vi "TDC_DAQV27_Paralled_muon.vi"(7 "address":string="192.168.10.20", 8 "error in (no error)":errorcluster, 9 "stop":bool, 10 "save data":bool=TRUE, 11 "SMA mode":bool=TRUE) -> (0 "error out 3":errorcluster, 2 "appended path":path=path "G:/tdc/2017/test_20250117_110508.dat", 3 "rate":dbl=15.409526451492772)   [LabVIEW 2017]
uses:
  <vilib>/Utility/file.llb/Write Delimited Spreadsheet (DBL).vi
  <vilib>/Utility/file.llb/Write Delimited Spreadsheet (I64).vi
panel:
  in  "timeot":dbl
  out "nearest integer value":dbl
  out "Out":u8=1 format="%.0x"
  out "fine 4":u64=243508331 format="%x"
  out "fine 3":u64=243508331 format="%x"
  out "channel number 2":u64 format="%x"
  out "substring 3":string
  out "fine 2":u64=243508331 format="%x"
  out "substring 2":string
  out "substring":string
  in  "gps":bool
  out "Year":string="2025"
  in  "factor":i32=128
  in  "displayCR":bool=TRUE
  in  "Counter Setting":dbl=100000.0 format="%#_13g"
  in  "replace dat":bool
  in  "append csv":bool=TRUE
  out "element":string
  out "fine":u64=416 format="%x"
  in  "UDP Config":bool=TRUE
  in  "data  path":path=path "G:/tdc/2017/data"
  out "cal 2":u64[](graph)
  in  "Thresholds (mV)":dbl[](array[numeric])=[580.0, 580.0, 580.0, 580.0, 600.0, 600.0, 600.0, 600.0, 580.0, 580.0, 600.0, 600.0, 600.0, 600.0, 600.0, 600.0, 580.0, 580.0, 600.0, 600.0, 600.0, 600.0, 600.0, 600.0, 580.0, 580.0, 600.0, 600.0, 600.0, 600.0, 600.0, 600.0, 600.0, 600.0, 600.0, 600.0, 600.0, 600.0, 600.0, 600.0, 600.0, 600.0, 600.0, 600.0, 600.0, 600.0, 600.0, 600.0, 600.0, 600.0, 600.0, 600.0, 600.0, 600.0, 600.0, 600.0, 600.0, 600.0, 600.0, 600.0, 600.0, 600.0, 600.0, 600.0]
  out "error out 2":errorcluster={"status"=TRUE, "code"=1, "source"="Dequeue Element in TDC_DAQV27_Paralled_muon.vi"}
  in  "display":bool=TRUE
  in  "Thresholds":dbl=8191.0
  in  "one key for threshold":bool=TRUE
  in  "RST":bool
  in  "通道数量":i32=128
  out "Cal Table":u32[](array[numeric])=[5700, 5700, 0, 0, 0, 0, 0, 0, 0, 0, 0, 0, 0, 0, 0, 0, 0, 0, 0, 0, 0, 0, 0, 0, 0, 0, 0, 0, 0, 0, 0, 0, 0, 0, 0, 0, 0, 0, 0, 0, 0, 0, 0, 0, 0, 0, 0, 0, 0, 0, 0, 0, 0, 0, 0, 0, 0, 0, 0, 0, 0, 0, 0, 0, 0, 0, 0, 0, 0, 0, 0, 0, 0, 0, 0, 0, 0, 0, 0, 0, 0, 0, 0, 0, 0, 0, 0, 0, 0, 0, 0, 0, 0, 0, 0, 0, 0, 0, 0, 0, 0, 0, 0, 0, 0, 0, 0, 0, 0, 0, 0, 0, 0, 0, 0, 0, 0, 0, 0, 0, 0, 0, 0, 0, 0, 0, 0, 0]
  in  "channel for cal":i32=1
  out "channel number":u64
  in  "bytes to read":i32=320
  out "Calibration Counter":i32=5699
  out "Event index":i32=97959
  out "cal":u32[](graph)=[0, 0, 0, 0, 0, 0, 0, 0, 0, 0, 0, 0, 0, 0, 0, 0, 0, 0, 0, 0, 0, 0, 0, 0, 0, 0, 0, 0, 0, 0, 0, 0, 0, 0, 0, 0, 0, 0, 0, 0, 0, 0, 0, 0, 0, 0, 0, 0, 0, 0, 0, 0, 0, 0, 0, 0, 0, 0, 0, 0, 0, 0, 0, 0, 0, 0, 0, 0, 0, 0, 0, 0, 0, 0, 0, 0, 0, 0, 0, 0, 0, 0, 0, 0, 0, 0, 0, 0, 0, 0, 0, 0, 0, 0, 0, 0, 0, 0, 0, 0, 0, 0, 0, 0, 0, 0, 0, 0, 0, 0, 0, 0, 0, 0, 0, 0, 0, 0, 0, 0, 0, 0, 0, 0, 0, 0, 0, 0, 0, 0, 0, 0, 0, 0, 0, 0, 0, 0, 0, 0, 0, 0, 0, 0, 0, 0, 0, 0, 0, 0, 0, 0, 0, 0, 0, 0, 0, 0, 0, 0, 0, 0, 0, 0, 0, 0, 0, 0, 0, 0, 0, 0, 0, 0, 0, 0, 0, 0, 0, 0, 0, 0, 0, 0, 0, 0, 0, 0, 0, 0, 0, 0, 0, 0, 0, 0, 0, 0, 0, 0, 0, 0, 0, 0, 0, 0, 0, 0, 0, 0, 0, 0, 0, 0, 0, 0, 0, 0, 0, 0, 0, 0, 0, 0, 0, 0, 0, 0, 15, 4, 8, 11, 19, 27, 12, 4, 29, 16, 7, 12, 3, 18, 8, 6, 6, 7, 3, 6, 4, 22, 0, 10, 13, 5, 6, 5, 8, 11, 3, 15, 13, 3, 10, 19, 16, 9, 12, 2, 11, 3, 19, 2, 4, 11, 12, 2, 0, 0, 0, 0, 0, 0, 0, 0, 0, 0, 0, 0, 0, 0, 0, 0, 0, 0, 0, 0, 0, 0, 0, 0, 17, 11, 8, 5, 6, 2, 5, 3, 1, 0, 0, 0, 0, 0, 1, 5, 3, 3, 2, 0, 0, 0, 0, 0, 0, 0, 1, 0, 2, 6, 6, 10, 9, 10, 15, 8, 9, 12, 7, 6, 9, 16, 13, 16, 23, 9, 3, 5, 21, 9, 15, 40, 30, 8, 12, 2, 10, 5, 7, 12, 16, 10, 5, 11, 11, 18, 7, 12, 15, 10, 9, 13, 17, 14, 4, 6, 15, 5, 7, 2, 9, 4, 9, 6, 26, 8, 5, 14, 10, 6, 6, 10, 16, 7, 12, 10, 20, 14, 25, 8, 1, 4, 2, 14, 3, 8, 6, 5, 10, 12, 3, 6, 5, 11, 8, 17, 3, 9, 5, 0, 0, 0, 0, 0, 0, 0, 0, 0, 0, 0, 0, 0, 0, 0, 0, 0, 0, 0, 0, 0, 0, 0, 0, 5, 6, 15, 12, 7, 9, 5, 10, 4, 1, 1, 0, 0, 0, 0, 0, 0, 0, 0, 0, 0, 0, 0, 0, 0, 0, 0, 0, 0, 0, 0, 0, 3, 3, 8, 10, 10, 4, 17, 8, 4, 3, 12, 10, 26, 10, 14, 9, 31, 11, 54, 7, 12, 8, 6, 14, 7, 7, 17, 29, 8, 22, 3, 11, 12, 7, 13, 7, 5, 8, 1, 10, 10, 14, 15, 11, 8, 13, 5, 9, 9, 15, 16, 22, 6, 5, 4, 9, 20, 32, 6, 2, 4, 14, 12, 6, 7, 15, 12, 13, 10, 18, 17, 11, 6, 6, 17, 14, 6, 7, 10, 4, 7, 7, 6, 20, 2, 6, 5, 16, 4, 5, 13, 15, 11, 10, 13, 1, 5, 12, 7, 17, 11, 9, 8, 9, 10, 12, 14, 14, 11, 10, 4, 3, 15, 13, 1, 15, 12, 4, 5, 8, 9, 4, 4, 3, 4, 15, 14, 14, 4, 6, 10, 5, 1, 12, 5, 3, 4, 3, 2, 7, 5, 10, 9, 16, 7, 16, 5, 6, 2, 7, 9, 5, 9, 19, 17, 4, 10, 4, 10, 9, 5, 12, 0, 0, 0, 0, 0, 0, 0, 5, 36, 14, 11, 7, 3, 4, 10, 10, 8, 14, 14, 7, 9, 3, 18, 3, 35, 19, 16, 14, 27, 7, 11, 13, 6, 0, 7, 2, 19, 17, 25, 11, 2, 6, 4, 3, 0, 0, 0, 0, 1, 0, 0, 0, 0, 0, 1, 9, 10, 4, 2, 4, 13, 26, 5, 14, 20, 20, 8, 2, 22, 5, 10, 30, 14, 8, 9, 14, 23, 17, 8, 9, 10, 7, 19, 26, 4, 13, 20, 7, 2, 14, 9, 5, 43, 8, 13, 8, 12, 10, 15, 42, 13, 24, 22, 21, 5, 7, 19, 5, 20, 10, 5, 10, 8, 10, 2, 14, 3, 36, 14, 9, 9, 10, 22, 14, 16, 12, 10, 12, 13, 13, 18, 15, 13, 21, 16, 5, 5, 4, 5, 3, 5, 16, 6, 11, 6, 7, 4, 21, 8, 6, 4, 1, 21, 6, 6, 10, 35, 26, 5, 7, 13, 14, 9, 7, 5, 15, 4, 5, 8, 4, 12, 10, 4, 6, 4, 5, 6, 25, 3, 10, 9, 7, 4, 7, 14, 6, 6, 15, 17, 23, 6, 6, 4, 5, 3, 11, 13, 23, 3, 8, 12, 2, 7, 13, 25, 18, 3, 10, 2, 7, 5, 4, 6, 12, 6, 31, 24, 12, 16, 12, 15, 11, 15, 2, 2, 2, 1, 5, 4, 14, 25, 9, 25, 4, 2, 4, 4, 11, 10, 7, 7, 5, 10, 12, 12, 2, 6, 12, 7, 4, 2, 0, 0, 0, 0, 0, 0, 0, 0, 0, 0, 0, 0, 0, 0, 0, 0, 0, 0, 0, 0, 0, 0, 0, 0, 0, 0, 0, 0, 0, 0, 0, 0, 0, 0, 0, 0, 0, 0, 0, 0, 0, 0, 0, 0, 0, 0, 0, 0, 0, 0, 0, 0, 0, 0, 0, 0, 0, 0, 0, 0, 0, 0, 0, 0, 0, 0, 0, 0, 0, 0, 0, 0, 0, 0, 0, 0, 0, 0, 0, 0, 0, 0, 0, 0, 0, 0, 0, 0, 0, 0, 0, 0, 0, 0, 0, 0, 0, 0, 0, 0, 0, 0, 0, 0, 0, 0, 0, 0, 0, 0, 0, 0, 0, 0, 0, 0, 0, 0, 0, 0, 0, 0, 0, 0, 0, 0, 0, 0, 0, 0, 0, 0, 0, 0, 0, 0, 0, 0, 0, 0, 0, 0, 0, 0, 0, 0, 0, 0, 0, 0, 0, 0, 0, 0, 0, 0, 0, 0, 0, 0, 0, 0, 0, 0, 0, 0, 0, 0, 0, 0, 0, 0, 0, 0, 0, 0, 0, 0, 0, 0, 0, 0, 0, 0, 0, 0, 0, 0, 0, 0, 0, 0, 0, 0, 0, 0, 0, 0, 0, 0, 0, 0, 0, 0, 0, 0, 0, 0, 0, 0, 0, 0, 0, 0, 0, 0, 0, 0, 0, 0, 0, 0, 0, 0, 0, 0, 0, 0, 0, 0, 0, 0, 0, 0, 0, 0, 0, 0, 0, 0, 0, 0, 0, 0, 0, 0, 0, 0, 0, 0, 0, 0, 0, 0, 0, 0, 0, 0, 0, 0, 0, 0, 0, 0, 0, 0, 0, 0, 0, 0, 0, 0, 0, 0, 0, 0, 0, 0, 0, 0, 0, 0, 0, 0, 0, 0, 0, 0, 0, 0, 0, 0, 0, 0, 0, 0, 0, 0, 0, 0, 0, 0, 0, 0, 0, 0, 0, 0, 0, 0, 0, 0, 0, 0, 0, 0, 0, 0, 0, 0, 0, 0, 0, 0, 0, 0, 0, 0, 0, 0, 0, 0, 0, 0, 0, 0, 0, 0, 0, 0, 0, 0, 0, 0, 0, 0, 0, 0, 0, 0, 0, 0, 0, 0, 0, 0, 0, 0, 0, 0, 0, 0, 0, 0, 0, 0, 0, 0, 0, 0, 0, 0, 0, 0, 0, 0, 0, 0, 0, 0, 0, 0, 0, 0, 0, 0, 0, 0, 0, 0, 0, 0, 0, 0, 0, 0, 0, 0, 0, 0, 0, 0, 0, 0, 0, 0, 0, 0, 0, 0, 0, 0, 0, 0, 0, 0, 0, 0, 0, 0, 0, 0, 0, 0, 0, 0, 0, 0, 0, 0, 0, 0, 0, 0, 0, 0, 0, 0, 0, 0, 0, 0, 0, 0, 0, 0, 0, 0, 0, 0, 0, 0, 0, 0, 0, 0, 0, 0, 0, 0, 0, 0, 0, 0, 0, 0, 0, 0, 0, 0, 0, 0, 0, 0, 0, 0, 0, 0, 0, 0, 0, 0, 0, 0, 0, 0, 0, 0, 0, 0, 0, 0, 0, 0, 0, 0, 0, 0, 0, 0, 0, 0, 0, 0, 0, 0, 0, 0, 0, 0, 0, 0, 0, 0, 0, 0, 0, 0, 0, 0, 0, 0, 0, 0, 0, 0, 0, 0, 0, 0, 0, 0, 0, 0, 0, 0, 0, 0, 0, 0, 0, 0, 0, 0, 0, 0, 0, 0, 0, 0, 0, 0, 0, 0, 0, 0, 0, 0, 0, 0, 0, 0, 0, 0, 0, 0, 0, 0, 0, 0, 0, 0, 0, 0, 0, 0, 0, 0, 0, 0, 0, 0, 0, 0, 0, 0, 0, 0, 0, 0, 0, 0, 0, 0, 0, 0, 0, 0, 0, 0, 0, 0, 0, 0, 0, 0, 0, 0, 0, 0, 0, 0, 0, 0, 0, 0, 0, 0, 0, 0, 0, 0, 0, 0, 0, 0, 0, 0, 0, 0, 0, 0, 0, 0, 0, 0, 0, 0, 0, 0, 0, 0, 0, 0, 0, 0, 0, 0, 0, 0, 0, 0, 0, 0, 0, 0, 0, 0, 0, 0, 0, 0, 0, 0, 0, 0, 0, 0, 0, 0, 0, 0, 0, 0, 0, 0, 0, 0, 0, 0, 0, 0, 0, 0, 0, 0, 0, 0, 0, 0, 0, 0, 0, 0, 0, 0, 0, 0, 0, 0, 0, 0, 0, 0, 0, 0, 0, 0, 0, 0, 0, 0, 0, 0, 0, 0, 0, 0, 0, 0, 0, 0, 0, 0, 0, 0, 0, 0, 0, 0, 0, 0, 0, 0, 0, 0, 0, 0, 0, 0, 0, 0, 0, 0, 0, 0, 0, 0, 0, 0, 0, 0, 0, 0, 0, 0, 0, 0, 0, 0, 0, 0, 0, 0, 0, 0, 0, 0, 0, 0, 0, 0, 0, 0, 0, 0, 0, 0, 0, 0, 0, 0, 0, 0, 0, 0, 0, 0, 0, 0, 0, 0, 0, 0, 0, 0, 0, 0, 0, 0, 0, 0, 0, 0, 0, 0, 0, 0, 0, 0, 0, 0, 0, 0, 0, 0, 0, 0, 0, 0, 0, 0, 0, 0, 0, 0, 0, 0, 0, 0, 0, 0, 0, 0, 0, 0, 0, 0, 0, 0, 0, 0, 0, 0, 0, 0, 0, 0, 0, 0, 0, 0, 0, 0, 0, 0, 0, 0, 0, 0, 0, 0, 0, 0, 0, 0, 0, 0, 0, 0, 0, 0, 0, 0, 0, 0, 0, 0, 0, 0, 0, 0, 0, 0, 0, 0, 0, 0, 0, 0, 0, 0, 0, 0, 0, 0, 0, 0, 0, 0, 0, 0, 0, 0, 0, 0, 0, 0, 0, 0, 0, 0, 0, 0, 0, 0, 0, 0, 0, 0, 0, 0, 0, 0, 0, 0, 0, 0, 0, 0, 0, 0, 0, 0, 0, 0, 0, 0, 0, 0, 0, 0, 0, 0, 0, 0, 0, 0, 0, 0, 0, 0, 0, 0, 0, 0, 0, 0, 0, 0, 0, 0, 0, 0, 0, 0, 0, 0, 0, 0, 0, 0, 0, 0, 0, 0, 0, 0, 0, 0, 0, 0, 0, 0, 0, 0, 0, 0, 0, 0, 0, 0, 0, 0, 0, 0, 0, 0, 0, 0, 0, 0, 0, 0, 0, 0, 0, 0, 0, 0, 0, 0, 0, 0, 0, 0, 0, 0, 0, 0, 0, 0, 0, 0, 0, 0, 0, 0, 0, 0, 0, 0, 0, 0, 0, 0, 0, 0, 0, 0, 0, 0, 0, 0, 0, 0, 0, 0, 0, 0, 0, 0, 0, 0, 0, 0, 0, 0, 0, 0, 0, 0, 0, 0, 0, 0, 0, 0, 0, 0, 0, 0, 0, 0, 0, 0, 0, 0, 0, 0, 0, 0, 0, 0, 0, 0, 0, 0, 0, 0, 0, 0, 0, 0, 0, 0, 0, 0, 0, 0, 0, 0, 0, 0, 0, 0, 0, 0, 0, 0, 0, 0, 0, 0, 0, 0, 0, 0, 0, 0, 0, 0, 0, 0, 0, 0, 0, 0, 0, 0, 0, 0, 0, 0, 0, 0, 0, 0, 0, 0, 0, 0, 0, 0, 0, 0, 0, 0, 0, 0, 0, 0, 0, 0, 0, 0, 0, 0, 0, 0]
  out "error out":errorcluster
  in  "filename":string="test"
  in  "Events":i32=110000 min=1
  in  "timeout (ms)":i32=10000
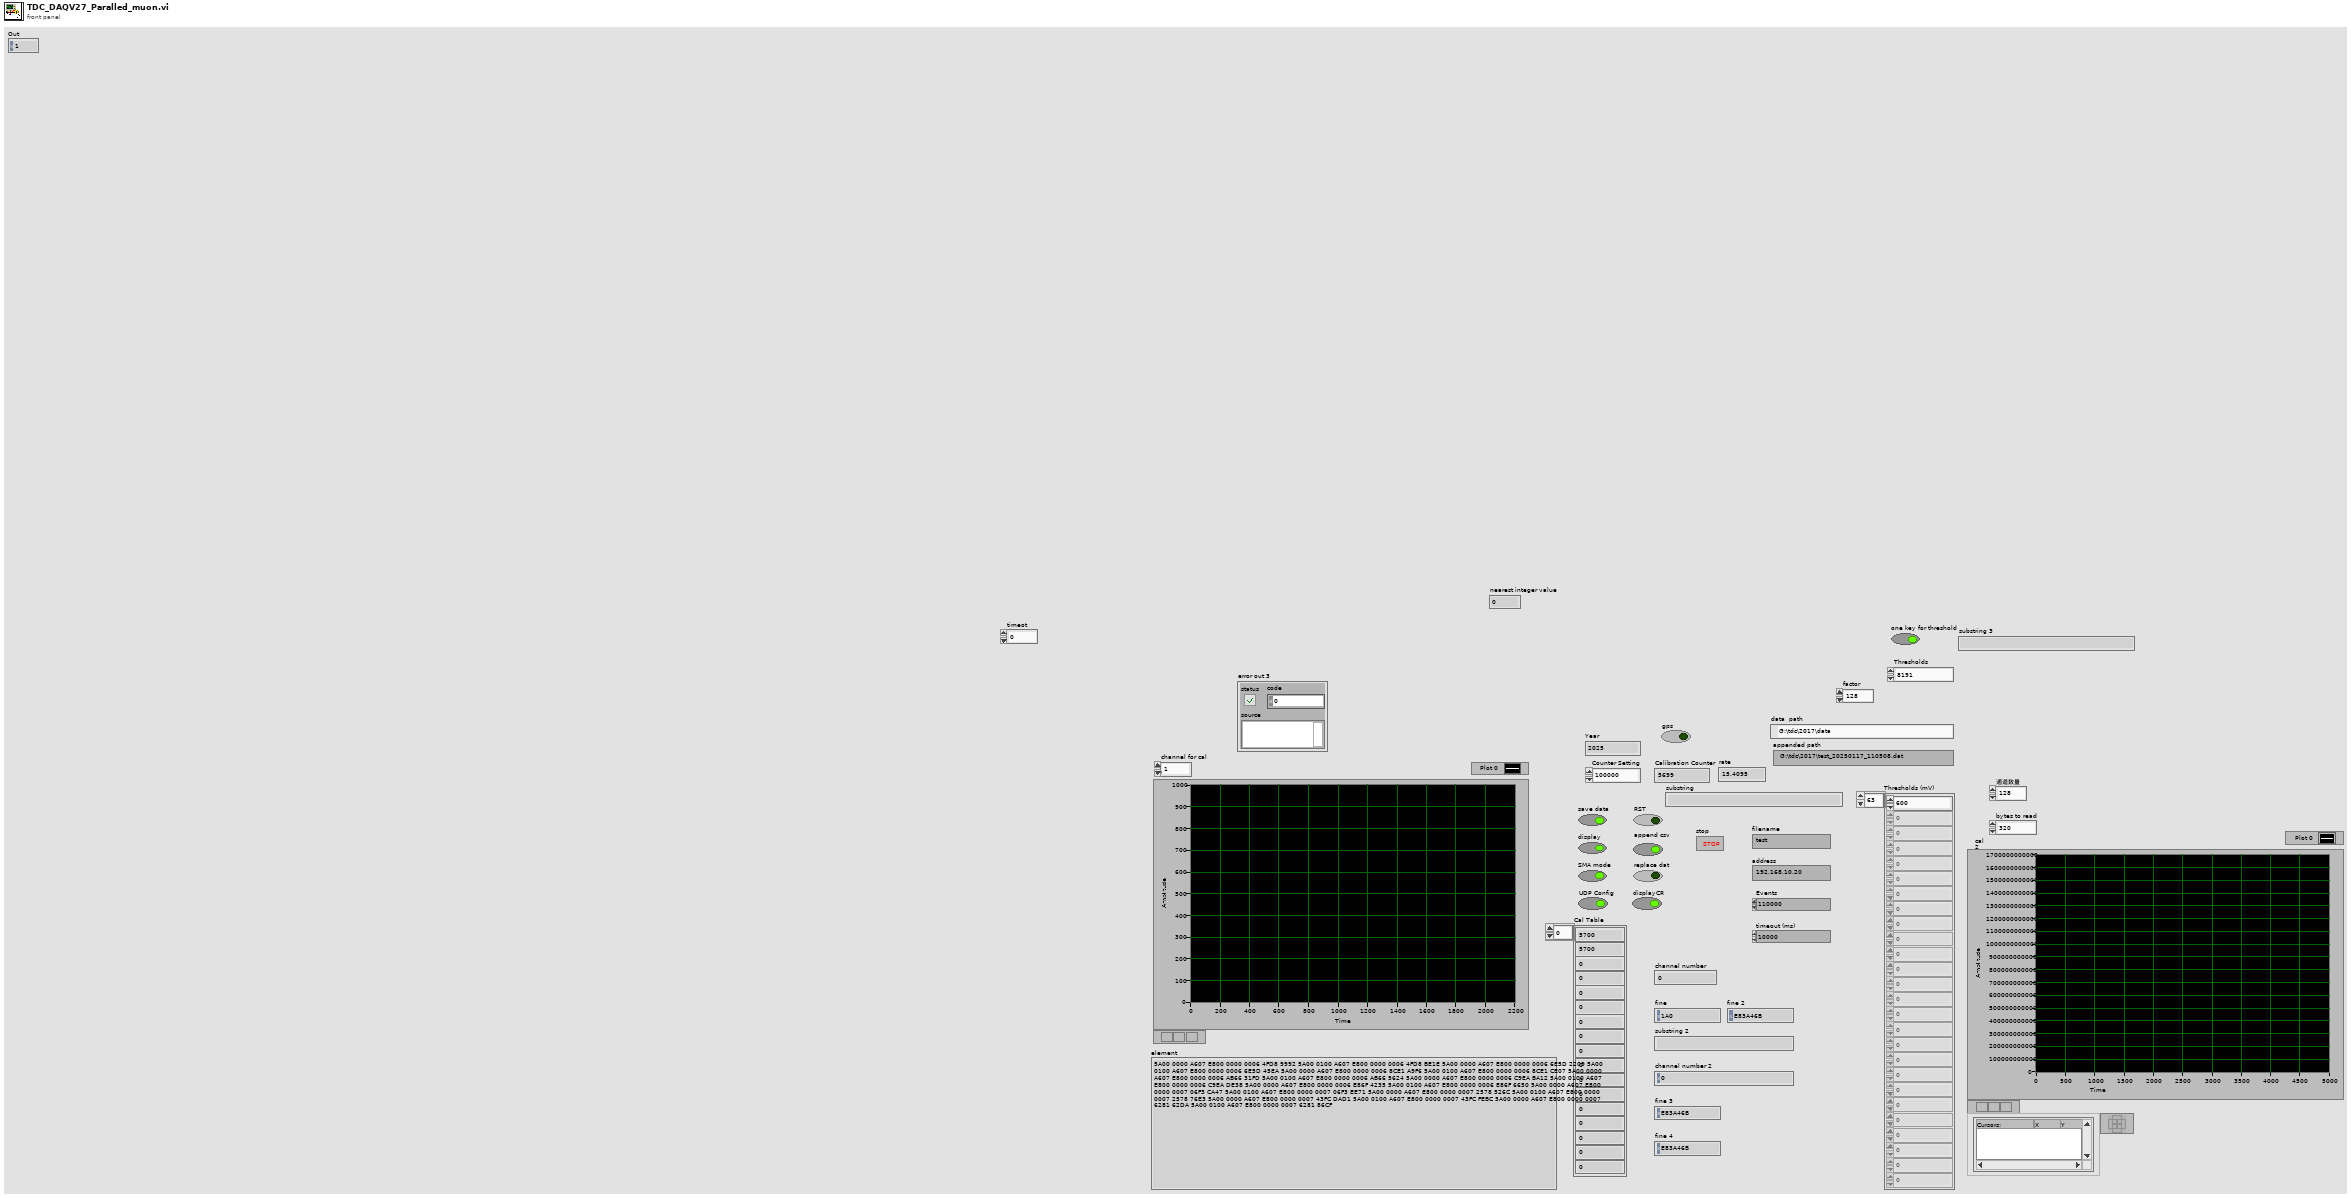
[diagram p1: front panel]
types:
  T1 = enum16{"open", "replace", "create", "open or create", "replace or create", "replace or create with confirmation"}
  T2 = enum16{"Standard", "Buffered", "CRLF", "Immediate"}
  T3 = enum16{"big-endian, network order", "native, host order", "little-endian"}
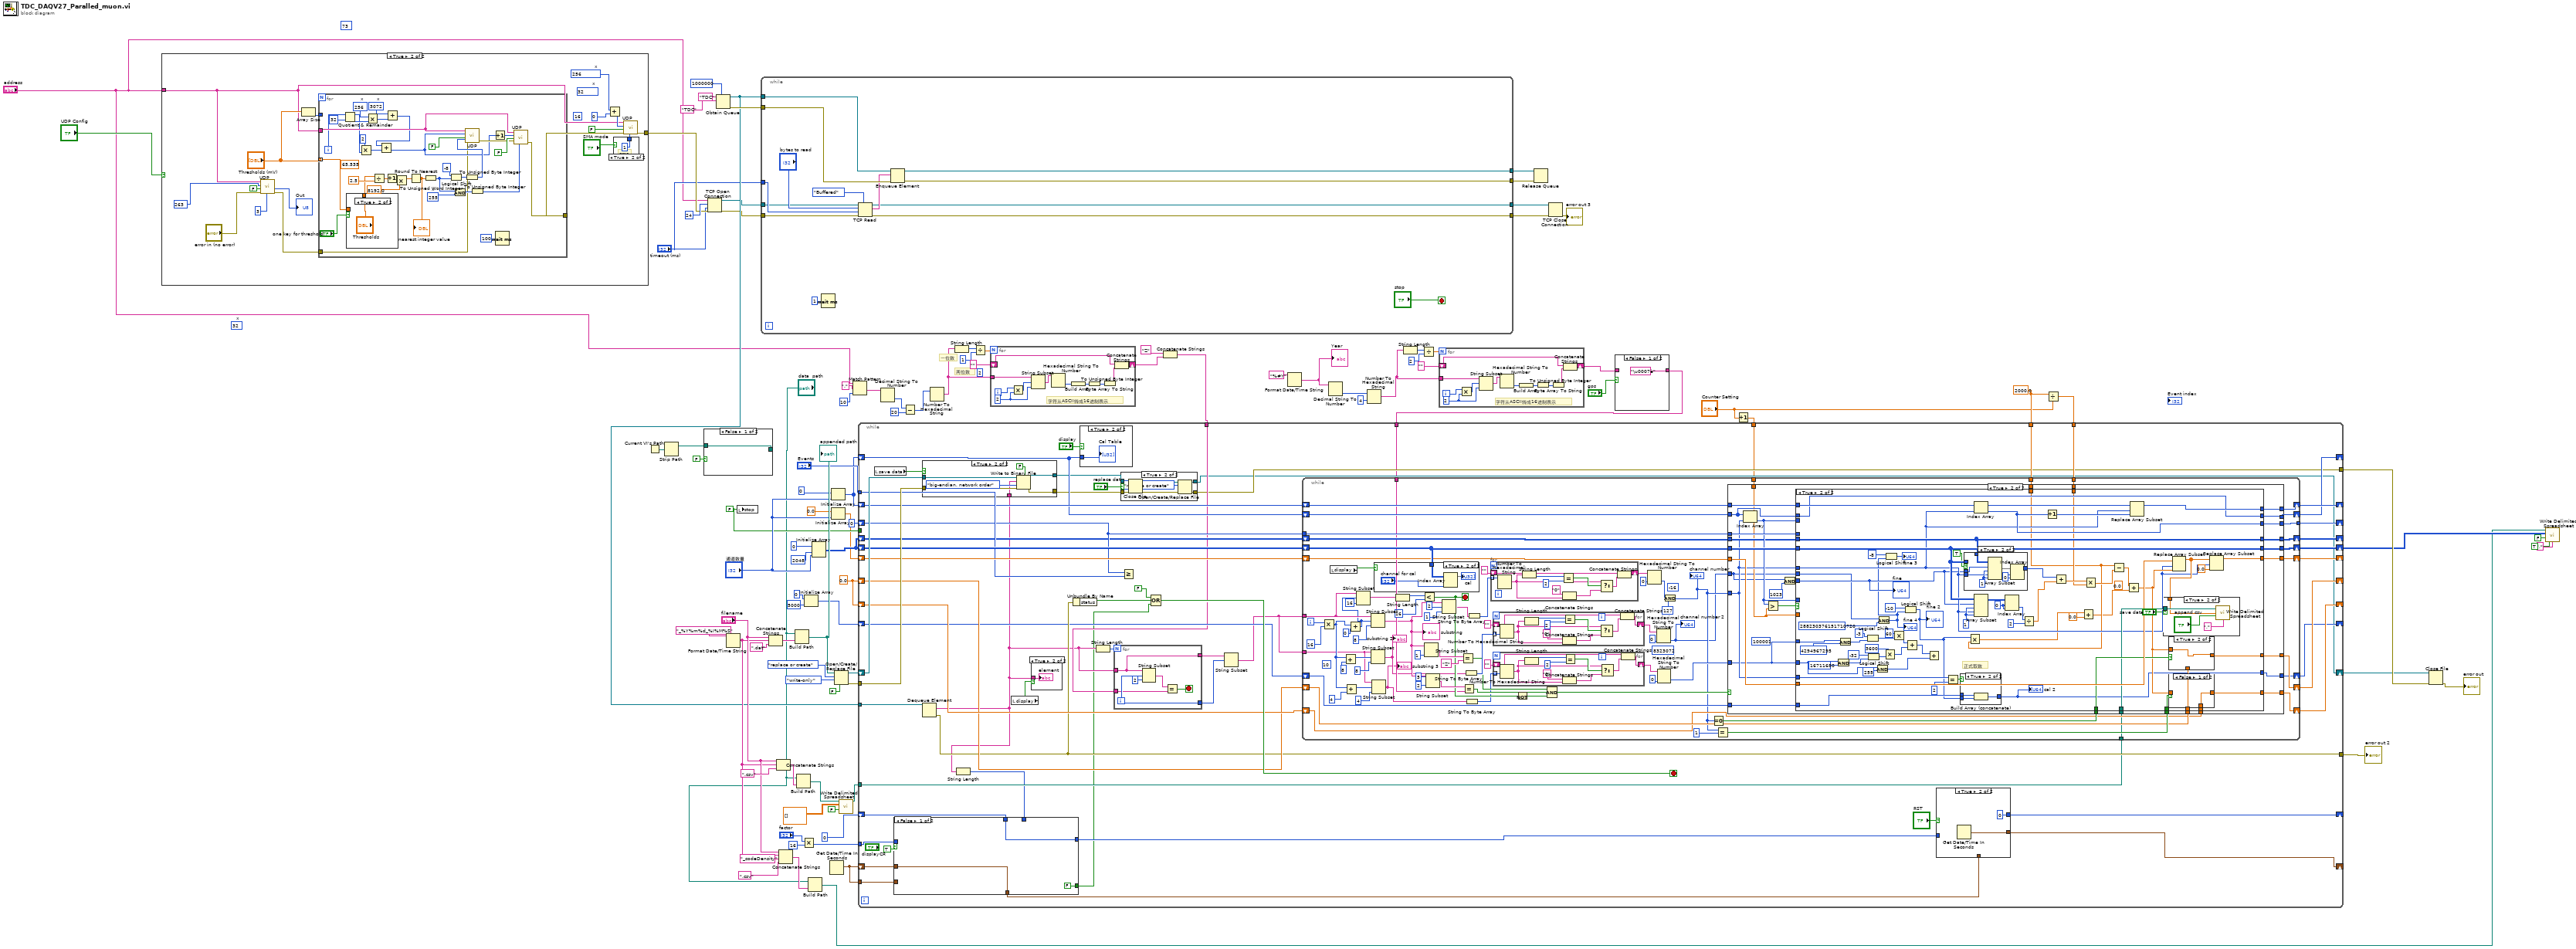
[diagram p0: block diagram]
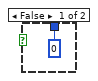
[diagram p4: hidden frame]
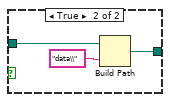
[diagram p6: hidden frame]
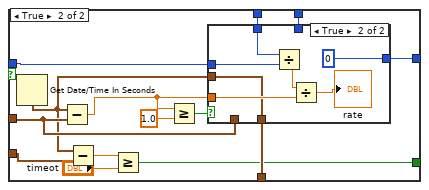
[diagram p10: hidden frame]
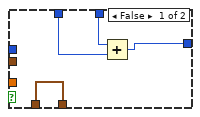
[diagram p11: hidden frame]
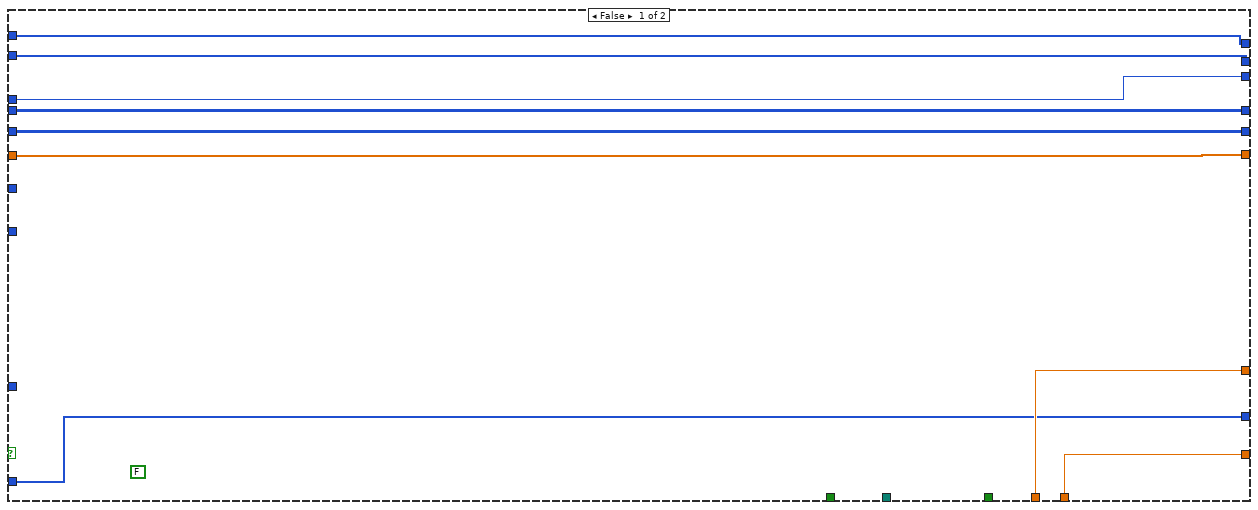
[diagram p15: hidden frame]
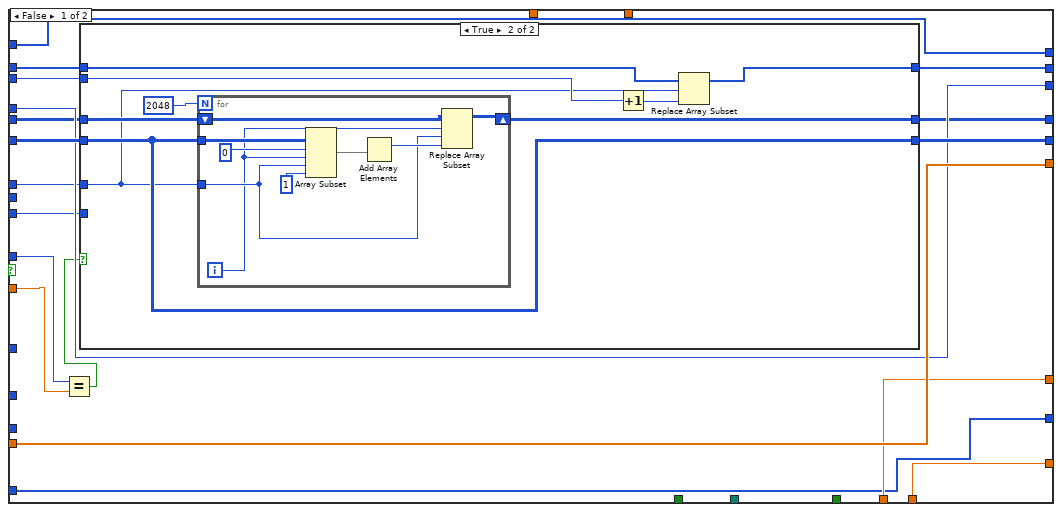
[diagram p16: hidden frame]
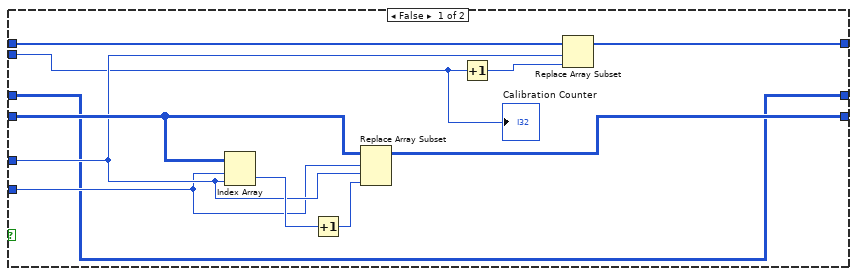
[diagram p17: hidden frame]
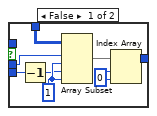
[diagram p20: hidden frame]
diagram:
  (unwired) u32 73 ("Address")
  (unwired) 2 ("y")
  w29 = 2000.0 ("x")
  (unwired) u16 32  # x
  w69 = FALSE ("stop")
  w78 = 0.0
  # "一位数"
  # "两位数"
  n1 = case shown="True" "UDP Config" {
    tunnel: "address" -> [_ w103]
    tunnel: [_ w115] -> w70
    frame False {
    }
    frame True {
      (unwired) u16 32  # x
      (unwired) u32 16 ("Address")
      w108 = u16 256  # x
      n2 = call "UDP.vi"("In"=u8 3, "error in (no error)"="error in (no error)", "Read (TRUE)"=FALSE, "Address"=u32 263, "IP address"=w103) -> ("error out"=w101:errorcluster, "Out"=→"Out":u8)  [unwired: 4 in]
      n3 = Array Size(array="Thresholds (mV)") -> (size(s)=w112:i32)
      n4 = for {
        tunnel: w103 -> [w149]
        tunnel: "Thresholds (mV)" -> [w136] mode=indexing
        tunnel: [w139] -> w116
        tunnel: w112 -> [_]
        tunnel: w101 -> [w123]
        i -> [w131]
        (unwired) 65.535 ("y")
        w132 = u16 3072  # x
        w133 = u16 256  # x
        w145 = u16 255  # x
        n5 = Quotient & Remainder(x=w131, y=32) -> (x-y*floor(x/y)=w125:i32, floor(x/y)=w134:i32)
        n6 = case shown="True" "one key for threshold" {
          tunnel: [w155 "Thresholds"] -> w137
          tunnel: w136 -> [w155 _]
          frame False {
          }
          frame True {
          }
        }
        n7 = Multiply(x=2, y=w125) -> (x*y=w126:i32)
        n8 = Multiply(x=w133, y=w134) -> (x*y=w128:i32)
        n9 = Divide(x=w137, y=2.5) -> (x/y=w152:dbl)
        n10 = Increment(x=w152) -> (x+1=w122:dbl)
        n11 = Add(x=w132, y=w128) -> (x+y=w127:i32)
        n12 = Add(x=w127, y=w126) -> (x+y=w130:i32)
        n13 = Multiply(x=w122, y=8192.0) -> (x*y=w121:dbl)
        n14 = Round To Nearest(number=w121) -> (nearest integer value=w150:dbl)
        "nearest integer value" <- w150
        n15 = To Unsigned Word Integer(number=w150) -> (unsigned 16bit integer=w141:u16)
        n16 = Logical Shift(y=i16 -8, x=w141) -> (x << y=w147:u16)
        n17 = And(x=w141, y=w145) -> (x .and. y?=w144:u16)
        n18 = To Unsigned Byte Integer(number=w147) -> (unsigned 8bit integer=w146:u8)
        n19 = call "UDP.vi"("In"=w146, "error in (no error)"=w123, "Read (TRUE)"=FALSE, "Address"=w130, "IP address"=w149) -> ("error out"=w140:errorcluster)  [unwired: 4 in, 1 out]
        n20 = To Unsigned Byte Integer(number=w144) -> (unsigned 8bit integer=w143:u8)
        n21 = Increment(x=w130) -> (x+1=w129:i32)
        n22 = Wait (ms)(milliseconds to wait=u32 100) -> ()  [unwired: 1 out]
        n23 = call "UDP.vi"("In"=w143, "error in (no error)"=w140, "Read (TRUE)"=FALSE, "Address"=w129, "IP address"=w149) -> ("error out"=w139:errorcluster)  [unwired: 4 in, 1 out]
      }
      n24 = Add(x=w108, y=u32 0 ("Address")) -> (x+y=w109:u32)
      n25 = case shown="True" "SMA mode" {
        tunnel: [u8 0 ("In") u8 1 ("In")] -> w114
        frame False {
        }
        frame True {
          # "sma"
        }
      }
      n26 = call "UDP.vi"("In"=w114, "error in (no error)"=w116, "Read (TRUE)"=FALSE, "Address"=w109, "IP address"=w103) -> ("error out"=w115:errorcluster)  [unwired: 4 in, 1 out]
    }
  }
  n27 = Current VI's Path() -> (path=w94:path)
  n28 = Strip Path(path=w94) -> (stripped path=w93:path)  [unwired: 1 out]
  n29 = case shown="False" FALSE {
    tunnel: w93 -> [w157 w159]
    tunnel: [w157 w158] -> _
    frame False {
    }
    frame True {
      n30 = Build Path(base path=w159, name or relative path="data\\") -> (appended path=w158:path)
    }
  }
  n31 = TCP Open Connection(address="address", remote port or service name=u16 24 ("port"), timeout ms (60000)="timeout (ms)", error in (no error)=w70) -> (connection ID=w53:refnum<k5>, error out=w54:errorcluster)  [unwired: 1 in]
  n32 = Obtain Queue(max queue size (-1, unlimited)=1000000, name (unnamed)="TDC", element data type="TDC" ("name (unnamed)")) -> (queue out=w55:refnum<queue>, error out=w56:errorcluster)  [unwired: 2 in, 1 out]
  n33 = Format Date/Time String(time format string (%c)="_%Y%m%d_%I%M%S") -> (date/time string=w67:string)  [unwired: 2 in]
  n34 = local write "stop"(w69) -> ()
  n35 = while {
    tunnel: w55 -> [w174]
    tunnel: w56 -> [w173]
    tunnel: w54 -> [w171]
    tunnel: "timeout (ms)" -> [w170]
    tunnel: w53 -> [w169]
    tunnel: [w167] -> w52
    tunnel: [w166] -> w51
    tunnel: [w164] -> w50
    tunnel: [w163] -> w49
    stop <- "stop" stop-if-true
    n36 = Wait (ms)(milliseconds to wait=u32 1) -> ()  [unwired: 1 out]
    n37 = TCP Read(connection ID=w169, bytes to read="bytes to read", error in (no error)=w171, 7:T2."Buffered" ("mode (standard)"), 9:w170) -> (connection ID out=w167:refnum<k5>, data out=w168:string, error out=w166:errorcluster)
    n38 = Enqueue Element(queue=w174, element=w168, error in (no error)=w173) -> (queue out=w164:refnum<queue>, error out=w163:errorcluster)  [unwired: 1 in, 1 out]
  }
  n39 = Concatenate Strings("filename", w67, ".dat") -> (w92:string)
  n40 = Concatenate Strings("filename", w67, ".csv") -> (w80:string)
  n41 = Concatenate Strings("filename", w67, "_codeDensity" ("string"), ".csv") -> (w64:string)
  n42 = Build Path(base path="data  path", name or relative path=w92) -> (appended path=w91:path)
  "appended path" <- w91
  n43 = Build Path(base path="data  path", name or relative path=w80) -> (appended path=w75:path)
  n44 = Multiply(x="factor", y=16) -> (x*y=w22:i32)
  n45 = Initialize Array(u32 0 ("element"), 5000 ("dimension size")) -> (w43:u32[])
  n46 = Build Path(base path="data  path", name or relative path=w64) -> (appended path=w61:path)
  n47 = Initialize Array(u32 0 ("element"), 2048 ("dimension size"), "通道数量") -> (w77:u32[][])
  n48 = Get Date/Time In Seconds() -> (seconds since 1Jan1904=w1:timestamp)
  n49 = Initialize Array(u32 0 ("element"), "通道数量") -> (w79:u32[])
  n50 = Initialize Array(0.0, "通道数量") -> (w45:dbl[])
  n51 = Open/Create/Replace File(file path (use dialog)=w91, operation (0:open)=T1."replace or create", access (0:read/write)=enum16{"read/write", "read-only", "write-only"}."write-only", disable buffering (F)=FALSE) -> (refnum out=w96:refnum<file>, error out=w95:errorcluster)  [unwired: 2 in, 1 out]
  n52 = call-poly <vilib>:"Write Delimited Spreadsheet.vi"("file path (dialog if empty)"=w75, "2D data"=dbl[][] [], "append to file? (new file:F)"=FALSE) -> ("new file path (Not A Path if cancelled)"=w74:path)  [unwired: 11 in, 1 out]
  n53 = Match Pattern(string="address", regular expression="." ("search string"), offset (0)=10) -> (after substring=w32:string)  [unwired: 3 out]
  n54 = Decimal String To Number(string=w32) -> (number=w6:i32)  [unwired: 2 in, 1 out]
  n55 = Subtract(x=w6, y=20) -> (x-y=w5:i32)
  n56 = Number To Hexadecimal String(2:w5) -> (0:w31:string)  [unwired: 1 in]
  n57 = String Length(string=w31) -> (length=w37:i32)
  n58 = Divide(x=w37, y=1) -> (x/y=w38:dbl)
  n59 = for {
    N: w38 -> [_]
    shift-right: [w185] -> w4
    shift-left: "" ("format string") -> [w184]
    tunnel: w31 -> [w175]
    i -> [w183]
    w177 = 2 ("y")
    # "字符从ASCII转成16进制表示"
    n60 = Multiply(x=w183, y=w177) -> (x*y=w176:i32)
    n61 = String Subset(string=w175, offset (0)=w176, length (rest)=w177) -> (substring=w178:string)
    n62 = Hexadecimal String To Number(string=w178) -> (number=w182:u32)  [unwired: 2 in, 1 out]
    n63 = Build Array(w182) -> (w181:u32[])
    n64 = To Unsigned Byte Integer(number=w181) -> (unsigned 8bit integer=w180:u8[])
    n65 = Byte Array To String(unsigned byte array=w180) -> (string=w179:string)
    n66 = Concatenate Strings(w184, w179) -> (w185:string)
  }
  n67 = Concatenate Strings("Z", w4) -> (w3:string)
  n68 = Format Date/Time String(time format string (%c)="%#Y") -> (date/time string=w18:string)  [unwired: 2 in]
  "Year" <- w18
  n69 = Decimal String To Number(string=w18) -> (number=w17:i32)  [unwired: 2 in, 1 out]
  n70 = Number To Hexadecimal String(1:i16 4 ("width (-)"), 2:w17) -> (0:w11:string)
  n71 = String Length(string=w11) -> (length=w13:i32)
  n72 = Divide(x=w13, y=2) -> (x/y=w14:dbl)
  n73 = for {
    N: w14 -> [_]
    shift-right: [w196] -> w10
    shift-left: "" ("format string") -> [w195]
    tunnel: w11 -> [w186]
    i -> [w194]
    w188 = 2 ("y")
    # "字符从ASCII转成16进制表示"
    n74 = Multiply(x=w194, y=w188) -> (x*y=w187:i32)
    n75 = String Subset(string=w186, offset (0)=w187, length (rest)=w188) -> (substring=w189:string)
    n76 = Hexadecimal String To Number(string=w189) -> (number=w193:u32)  [unwired: 2 in, 1 out]
    n77 = Build Array(w193) -> (w192:u32[])
    n78 = To Unsigned Byte Integer(number=w192) -> (unsigned 8bit integer=w191:u8[])
    n79 = Byte Array To String(unsigned byte array=w191) -> (string=w190:string)
    n80 = Concatenate Strings(w195, w190) -> (w196:string)
  }
  n81 = Release Queue(queue=w50, error in (no error)=w49) -> ()  [unwired: 1 in, 3 out]
  n82 = TCP Close Connection(connection ID=w52, error in (no error)=w51) -> (error out=→"error out 3":errorcluster)  [unwired: 1 in, 1 out]
  n83 = case shown="False" "gps" {
    tunnel: w10 -> [_ w198]
    tunnel: ["\u0007è" ("format string") w198] -> w9
    frame False {
    }
    frame True {
    }
  }
  n84 = Increment(x="Counter Setting") -> (x+1=w25:dbl)
  n85 = Divide(x=w29, y="Counter Setting") -> (x/y=w28:dbl)
  n86 = while {
    tunnel: w95 -> [w255]
    tunnel: [w229] -> w48
    tunnel: [w213] -> w88
    shift-right: [w252] -> w62
    shift-left: w77 -> [w253]
    shift-right: [w238] -> _
    shift-left: w45 -> [w251]
    tunnel: "Events" -> [w249]
    shift-right: [w248] -> _
    shift-left: w79 -> [w247]
    shift-right: [w246] -> _
    shift-left: u32 0 ("element") -> [w245]
    shift-right: [w244] -> _
    shift-left: w79 -> [w231]
    shift-right: [w243] -> _
    shift-left: w78 -> [w240]
    shift-right: [w242] -> _
    shift-left: w78 -> [w241]
    shift-right: [w233] -> _
    shift-left: w77 -> [w239]
    tunnel: w74 -> [w225]
    shift-right: [w237] -> _
    shift-left: 0 -> [w207]
    shift-right: [w235] -> _
    shift-left: w1 -> [w234]
    tunnel: w69 -> [_]
    tunnel: w55 -> [w230]
    shift-right: [w226] -> _
    shift-left: w43 -> [w227]
    tunnel: w3 -> [w221]
    tunnel: w29 -> [w219]
    tunnel: w28 -> [w218]
    shift-right: [w212] -> w27
    shift-left: w96 -> [w254]
    tunnel: w25 -> [w211]
    tunnel: w22 -> [w204]
    tunnel: w9 -> [w201]
    tunnel: w1 -> [w200]
    stop <- w250 stop-if-true
    n87 = local read "save data"() -> (w206:bool)
    n88 = Dequeue Element(queue=w230) -> (element=w217:string, error out=w229:errorcluster)  [unwired: 2 in, 2 out]
    n89 = case shown="True" w206 {
      tunnel: w255 -> [w257 w265]
      tunnel: w254 -> [w258 w264]
      tunnel: w217 -> [_ w261]
      tunnel: [w258 w260] -> w216
      tunnel: [w257 w259] -> w214
      frame False {
      }
      frame True {
        n90 = Write to Binary File(file (use dialog)=w264, data=w261, error in=w265, 5:FALSE ("prepend array or string size? (T)"), 9:T3."big-endian, network order" ("byte order (0:big-endian, network order)")) -> (refnum out=w260:refnum<file>, error out=w259:errorcluster)  [unwired: 1 in, 1 out]
      }
    }
    n91 = String Length(string=w217) -> (length=w208:i32)
    n92 = case shown="False" TRUE {
      tunnel: w234 -> [w283 w293]
      tunnel: [w283 w294] -> w210
      tunnel: w207 -> [w282 w292]
      tunnel: w208 -> [_ w291]
      tunnel: [w282 w290] -> w209
      tunnel: w204 -> [_ w289]
      tunnel: w200 -> [_ w287]
      tunnel: [FALSE w284] -> w199
      frame False {
      }
      frame True {
        n93 = Get Date/Time In Seconds() -> (seconds since 1Jan1904=w288:timestamp)
        n94 = Subtract(x=w288, y=w293) -> (x-y=w296:dbl)
        n95 = Subtract(x=w288, y=w287) -> (x-y=w286:dbl)
        n96 = Greater Or Equal?(x=w286, y="timeot") -> (x >= y?=w284:bool)
        n97 = Greater Or Equal?(x=w296, y=1.0) -> (x >= y?=w297:bool)
        n98 = case shown="True" w297 {
          tunnel: w296 -> [_ w308]
          tunnel: w288 -> [_ w306]
          tunnel: [w301 w306] -> w294
          tunnel: w293 -> [w301 _]
          tunnel: w292 -> [w300 w303]
          tunnel: w291 -> [w299 _]
          tunnel: [w298 0] -> w290
          tunnel: w289 -> [_ w302]
          frame False {
            n99 = Add(x=w299, y=w300) -> (x+y=w298:i32)
          }
          frame True {
            n100 = Divide(x=w303, y=w302) -> (x/y=w305:dbl)
            n101 = Divide(x=w305, y=w308) -> (x/y=→"rate":dbl)
          }
        }
      }
    }
    n102 = local read "display"() -> (w205:bool)
    n103 = case shown="True" w205 {
      tunnel: w217 -> [_ w256]
      frame False {
      }
      frame True {
        "element" <- w256
      }
    }
    n104 = Unbundle By Name(w229) -> ("status"=w228:bool)
    n105 = case shown="True" "display" {
      tunnel: w231 -> [_ w309]
      frame False {
      }
      frame True {
        "Cal Table" <- w309
      }
    }
    n106 = String Length(string=w217) -> (length=w224:i32)
    n107 = for {
      N: w224 -> [_]
      tunnel: w217 -> [w277]
      tunnel: [w277] -> w223
      tunnel: [w276] -> w222
      tunnel: w221 -> [w275]
      i -> [w276]
      stop <- w278 stop-if-true
      n108 = String Subset(string=w277, offset (0)=w276, length (rest)=2 ("length (rest)")) -> (substring=w279:string)
      n109 = Equal?(x=w279, y=w275) -> (x = y?=w278:bool)
    }
    n110 = case shown="True" "replace dat" {
      tunnel: w216 -> [w267 w273]
      tunnel: [w267 w272] -> w212
      tunnel: w214 -> [w266 w269]
      tunnel: [w266 w268] -> w213
      frame False {
      }
      frame True {
        n111 = Close File(refnum=w273, error in=w269) -> (path=w274:path, error out=w270:errorcluster)
        n112 = Open/Create/Replace File(file path (use dialog)=w274, error in=w270, operation (0:open)=T1."replace or create") -> (refnum out=w272:refnum<file>, error out=w268:errorcluster)  [unwired: 3 in, 1 out]
      }
    }
    n113 = Greater Or Equal?(x=w245, y=w249) -> ()  [unwired: 1 out]
    n114 = Compound Arithmetic op=OR(FALSE ("x"), w228, w199) -> (w250:bool)
    n115 = String Subset(string=w223, offset (0)=w222) -> (substring=w202:string)  [unwired: 1 in]
    n116 = while {
      tunnel: w202 -> [w341]
      shift-right: [w388] -> w252
      shift-left: w253 -> [w386]
      shift-right: [w384] -> w238
      shift-left: w251 -> [w385]
      shift-right: [w381] -> w248
      shift-left: w247 -> [w380]
      tunnel: [w379] -> w246
      tunnel: w245 -> [w378]
      shift-right: [w376] -> w244
      shift-left: w231 -> [w377]
      shift-right: [w372] -> w243
      shift-left: w240 -> [w370]
      shift-right: [w368] -> w242
      shift-left: w241 -> [w369]
      tunnel: w225 -> [w367]
      shift-right: [w366] -> w233
      shift-left: w239 -> [w335]
      shift-right: [w363] -> w226
      shift-left: w227 -> [w364]
      tunnel: w202 -> [w328]
      tunnel: w219 -> [w343]
      tunnel: w218 -> [w342]
      tunnel: w211 -> [w334]
      tunnel: w201 -> [w322]
      i -> [w389]
      stop <- w337 stop-if-true
      (unwired) 10 ("length (rest)")
      (unwired) u64 8323072 ("port")
      (unwired) i16 -16 ("y")
      n117 = Multiply(x=w389, y=16 ("length (rest)")) -> (x*y=w329:i32)
      n118 = local read "display"() -> (w365:bool)
      n119 = Add(x=w329, y=8 ("length (rest)")) -> (x+y=w355:i32)
      n120 = Add(x=w329, y=4 ("length (rest)")) -> (x+y=w331:i32)
      n121 = Add(x=w329, y=0 ("length (rest)")) -> (x+y=w340:i32)
      n122 = String Subset(string=w341, offset (0)=w340, length (rest)=16 ("y")) -> (substring=w338:string)
      n123 = String Subset(string=w341, offset (0)=w340, length (rest)=8 ("length (rest)")) -> (substring=w320:string)
      "substring" <- w320
      n124 = String Subset(string=w328, offset (0)=w355, length (rest)=8 ("length (rest)")) -> (substring=w316:string)
      "substring 2" <- w316
      n125 = String Subset(string=w328, offset (0)=w331, length (rest)=4 ("length (rest)")) -> (substring=w315:string)
      "substring 3" <- w315
      n126 = case shown="True" w365 {
        tunnel: w386 -> [_ w415]
        frame False {
        }
        frame True {
          n127 = Index Array(array=w415, index (col)="channel for cal") -> (element=→"cal":u32[])  [unwired: 1 in]
        }
      }
      n128 = String Length(string=w338) -> (length=w383:i32)
      n129 = Less?(x=w383, y=16) -> (x < y?=w337:bool)
      n130 = String Subset(string=w320, length (rest)=1 ("length (rest)")) -> (substring=w360:string)  [unwired: 1 in]
      n131 = String Subset(string=w320, offset (0)=5, length (rest)=2 ("length (rest)")) -> (substring=w344:string)
      n132 = String Subset(string=w320, offset (0)=2, length (rest)=1 ("length (rest)")) -> (substring=w318:string)
      n133 = Equal?(x=w360, y="Z" ("format string")) -> (x = y?=w346:bool)
      n134 = Equal?(x=w344, y=w322) -> (x = y?=w345:bool)
      n135 = String To Byte Array(string=w316) -> (unsigned byte array=w352:u8[])
      n136 = String To Byte Array(string=w315) -> (unsigned byte array=w324:u8[])
      n137 = String To Byte Array(string=w318) -> (unsigned byte array=w391:u8[])
      n138 = for {
        shift-right: [w605] -> w349
        shift-left: "" ("format string") -> [w602]
        tunnel: w391 -> [w606] mode=indexing
        n139 = Number To Hexadecimal String(2:w606) -> (0:w598:string)  [unwired: 1 in]
        n140 = String Length(string=w598) -> (length=w604:i32)
        n141 = Equal?(x=w604, y=2) -> (x = y?=w601:bool)
        n142 = Concatenate Strings("0" ("format string"), w598) -> (w600:string)
        n143 = Select(t=w598, s=w601, f=w600) -> (s? t:f=w597:string)
        n144 = Concatenate Strings(w602, w597) -> (w605:string)
      }
      n145 = for {
        shift-right: [w411] -> w350
        shift-left: "" ("format string") -> [w403]
        tunnel: w352 -> [w412] mode=indexing
        n146 = Number To Hexadecimal String(2:w412) -> (0:w405:string)  [unwired: 1 in]
        n147 = String Length(string=w405) -> (length=w410:i32)
        n148 = Concatenate Strings("0" ("format string"), w405) -> (w407:string)
        n149 = Equal?(x=w410, y=2) -> (x = y?=w408:bool)
        n150 = Select(t=w405, s=w408, f=w407) -> (s? t:f=w404:string)
        n151 = Concatenate Strings(w403, w404) -> (w411:string)
      }
      n152 = for {
        shift-right: [w401] -> w327
        shift-left: "" ("format string") -> [w393]
        tunnel: w324 -> [w402] mode=indexing
        n153 = Number To Hexadecimal String(2:w402) -> (0:w395:string)  [unwired: 1 in]
        n154 = String Length(string=w395) -> (length=w400:i32)
        n155 = Concatenate Strings("0" ("format string"), w395) -> (w397:string)
        n156 = Equal?(x=w400, y=2) -> (x = y?=w398:bool)
        n157 = Select(t=w395, s=w398, f=w397) -> (s? t:f=w394:string)
        n158 = Concatenate Strings(w393, w394) -> (w401:string)
      }
      n159 = Not(x=w337) -> (.not. x?=w336:bool)
      n160 = Compound Arithmetic op=AND(w346, w345, w336) -> (w358:bool)
      n161 = Hexadecimal String To Number(string=w349, default (0uL)=u64 0 ("default (0 U32)")) -> (number=w387:u64)  [unwired: 1 in, 1 out]
      n162 = Hexadecimal String To Number(string=w350, default (0uL)=u64 0 ("default (0 U32)")) -> (number=w314:u64)  [unwired: 1 in, 1 out]
      "channel number 2" <- w314
      n163 = Hexadecimal String To Number(string=w327, default (0uL)=u64 0 ("default (0 U32)")) -> (number=w323:u64)  [unwired: 1 in, 1 out]
      n164 = And(x=w387, y=u64 127 ("port")) -> (x .and. y?=w317:u64)
      "channel number" <- w317
      n165 = Equal To 0?(x=w317) -> (x = 0?=w373:bool)
      n166 = Equal?(x=w317, y=u64 1) -> (x = y?=w371:bool)
      n167 = case shown="True" w358 {
        tunnel: w314 -> [_ w425]
        tunnel: w378 -> [w421 w446]
        tunnel: w386 -> [w424 w455]
        tunnel: [w424 w454] -> w388
        tunnel: [w423 w451] -> w384
        tunnel: w385 -> [w423 w450]
        tunnel: w317 -> [_ w430]
        tunnel: w380 -> [w422 w449]
        tunnel: [w422 w448] -> w381
        tunnel: [w421 w447] -> w379
        tunnel: w377 -> [w420 w445]
        tunnel: [w420 w444] -> w376
        tunnel: w373 -> [_ w443]
        tunnel: w370 -> [w419 w442]
        tunnel: [w419 w441] -> w372
        tunnel: w371 -> [_ w440]
        tunnel: w369 -> [w418 w439]
        tunnel: [w418 w438] -> w368
        tunnel: w335 -> [w417 w436]
        tunnel: [w417 w435] -> w366
        tunnel: w367 -> [_ w434]
        tunnel: w364 -> [w416 w432]
        tunnel: [w416 w431] -> w363
        tunnel: w343 -> [_ w429]
        tunnel: w342 -> [_ w428]
        tunnel: w334 -> [_ w427]
        tunnel: w323 -> [_ w426]
        frame False {
          (unwired) FALSE
        }
        frame True {
          (unwired) 100001 ("y")
          n168 = Index Array(array=w445, index=w430) -> (element=w437:u32)
          n169 = Greater?(x=w437, y=w427) -> (0:w433:bool)
          n170 = And(x=w425, y=u64 1023 ("port")) -> (x .and. y?=w452:u64)
          n171 = case shown="True" w433 {
            tunnel: w455 -> [w473 w557]
            tunnel: [w472 w557] -> w454
            tunnel: w452 -> [w464 w507]
            tunnel: [w471 w541] -> w451
            tunnel: w450 -> [w471 w564]
            tunnel: w446 -> [w469 _]
            tunnel: w430 -> [w467 w539]
            tunnel: w449 -> [w470 w563]
            tunnel: [w470 w562] -> w448
            tunnel: [w469 w560] -> w447
            tunnel: w437 -> [w465 _]
            tunnel: w445 -> [w468 w559]
            tunnel: [w466 w559] -> w444
            tunnel: w443 -> [_ w552]
            tunnel: w442 -> [w463 w551]
            tunnel: [w463 w550] -> w441
            tunnel: w440 -> [_ w549]
            tunnel: w439 -> [w462 w548]
            tunnel: [w462 w547] -> w438
            tunnel: w437 -> [w460 _]
            tunnel: w427 -> [w457 _]
            tunnel: w436 -> [w459 w543]
            tunnel: [w458 w543] -> w435
            tunnel: w434 -> [_ w542]
            tunnel: w432 -> [w456 w536]
            tunnel: [w456 w535] -> w431
            tunnel: w430 -> [_ w532]
            tunnel: w429 -> [_ w530]
            tunnel: w428 -> [_ w531]
            tunnel: w426 -> [_ w525]
            tunnel: w426 -> [_ w514]
            tunnel: w425 -> [_ w504]
            frame False {
              n172 = Equal?(x=w460, y=w457) -> (x = y?=w461:bool)
              n173 = case shown="True" w461 {
                tunnel: w473 -> [w484 w490]
                tunnel: [w482 w490] -> w472
                tunnel: w468 -> [w480 w488]
                tunnel: w467 -> [w479 w485]
                tunnel: [w477 w487] -> w466
                tunnel: w465 -> [w476 w486]
                tunnel: w464 -> [w475 _]
                tunnel: w459 -> [w474 w492]
                tunnel: [w474 w491] -> w458
                frame False {
                  n174 = Index Array(array=w484, index (row)=w475, index (col)=w479) -> (element=w483:u32)
                  n175 = Increment(x=w483) -> (x+1=w481:u32)
                  n176 = Replace Array Subset(array=w484, new element=w481, index (row)=w475, index (col)=w479) -> (w482:u32[][])
                  n177 = Increment(x=w476) -> (x+1=w478:u32)
                  n178 = Replace Array Subset(array=w480, new element=w478, index=w479) -> (w477:u32[])
                  "Calibration Counter" <- w476
                }
                frame True {
                  n179 = for {
                    N: 2048 -> [_]
                    tunnel: w490 -> [w502]
                    tunnel: w485 -> [w495]
                    shift-right: [w497] -> w491
                    shift-left: w492 -> [w498]
                    i -> [w494]
                    n180 = Array Subset(array=w502, index (row)=0 ("索引"), length (row)=w494, index (col)=w495, length (col)=1 ("长度")) -> (w499:u32[][])
                    n181 = Add Array Elements(numeric array=w499) -> (sum=w496:u32)
                    n182 = Replace Array Subset(array=w498, new element=w496, index (row)=w494, index (col)=w495) -> (w497:u32[][])
                  }
                  n183 = Increment(x=w486) -> (x+1=w489:u32)
                  n184 = Replace Array Subset(array=w488, new element=w489, index=w485) -> (w487:u32[])
                }
              }
            }
            frame True {
              (unwired) 0.0 ("x")
              w554 = 0 ("索引 (行)")
              w556 = 1 ("长度")
              # "正式取数"
              n185 = And(x=w514, y=u64 16711680 ("port")) -> (x .and. y?=w522:u64)
              n186 = And(x=w525, y=u64 4294967295 ("port")) -> (x .and. y?=w528:u64)
              n187 = Logical Shift(y=i16 -3, x=w528) -> (x << y=w509:u64)
              n188 = Logical Shift(y=i16 -32, x=w522) -> (x << y=w521:u64)
              n189 = And(x=w514, y=u64 255 ("port")) -> (x .and. y?=w513:u64)
              n190 = And(x=w504, y=u64 288230376151710720 ("port")) -> (x .and. y?=w503:u64)
              "fine 4" <- w503
              n191 = Multiply(x=u64 3600, y=w521) -> (x*y=w517:u64)
              n192 = Logical Shift(y=i16 -8, x=w503) -> (x << y=→"fine 3":u64)
              n193 = Multiply(x=u64 60, y=w509) -> (x*y=w518:u64)
              n194 = Logical Shift(y=i16 -10, x=w503) -> (x << y=w508:u64)
              "fine 2" <- w508
              n195 = Add(x=w518, y=w517) -> (x+y=w516:u64)
              n196 = Add(x=w516, y=w513) -> ()  [unwired: 1 out]
              n197 = Equal?(x=w532, y=u32 2) -> (x = y?=w534:bool)
              n198 = case shown="True" w534 {
                tunnel: w536 -> [w570 w573]
                tunnel: w508 -> [_ w572]
                tunnel: [w570 w571] -> w535
                frame False {
                }
                frame True {
                  n199 = Build Array (concatenate)(w573, w572) -> (w571:u64[])
                }
              }
              "cal 2" <- w535
              n200 = case shown="True" TRUE {
                tunnel: [w580 w588] -> w566
                tunnel: w557 -> [_ _]
                tunnel: w539 -> [w585 w586]
                tunnel: w507 -> [w583 w591]
                tunnel: w543 -> [w584 w592]
                frame False {
                  w579 = 0 ("index (row)")
                  w582 = 1 ("长度")
                  n201 = Decrement(x=w585) -> (x-1=w578:u64)
                  n202 = Array Subset(array=w584, index (row)=w583, length (row)=w582, index (col)=w578, length (col)=w582) -> (w581:u32[][])
                  n203 = Index Array(array=w581, index (row)=w579, index (col)=w579) -> (element=w580:u32)
                }
                frame True {
                  w587 = 0 ("index (row)")
                  w590 = 1 ("长度")
                  n204 = Array Subset(array=w592, index (row)=w591, length (row)=w590, index (col)=w586, length (col)=w590) -> (w589:u32[][])
                  n205 = Index Array(array=w589, index (row)=w587, index (col)=w587) -> (element=w588:u32)
                }
              }
              n206 = Multiply(x=w508, y=w530) -> (x*y=w512:dbl)
              n207 = Index Array(array=w563, index=w539) -> (element=w560:u32)
              n208 = Array Subset(array=w557, index (row)=w507, length (row)=w556, index (col)=w539, length (col)=w556) -> (w555:u32[][])
              n209 = Index Array(array=w555, index (row)=w554, index (col)=w554) -> (element=w553:u32)
              n210 = Divide(x=w553, y=u32 2) -> (x/y=w558:dbl)
              n211 = Increment(x=w560) -> (x+1=w561:u32)
              n212 = Add(x=w566, y=w558) -> (x+y=w565:dbl)
              n213 = Add(x=w512, y=0.0) -> (x+y=w511:dbl)
              n214 = Multiply(x=w565, y=w531) -> (x*y=w545:dbl)
              n215 = Subtract(x=w530, y=w545) -> (x-y=w529:dbl)
              n216 = Add(x=w529, y=w511) -> (x+y=w546:dbl)
              n217 = Replace Array Subset(array=w563, new element=w561, index=w539) -> (w562:u32[])
              n218 = case shown="True" w552 {
                tunnel: w546 -> [_ w596]
                tunnel: [w595 w596] -> w550
                tunnel: w551 -> [w595 _]
                frame False {
                }
                frame True {
                }
              }
              n219 = case shown="False" w549 {
                tunnel: [w593 w594] -> w547
                tunnel: w548 -> [w593 _]
                tunnel: w546 -> [_ w594]
                frame False {
                }
                frame True {
                }
              }
              n220 = Replace Array Subset(array=w564, new element=w546, index=w539) -> (w540:dbl[])
              n221 = case shown="True" "save data" {
                tunnel: w542 -> [_ w577]
                tunnel: w540 -> [_ w575]
                frame False {
                }
                frame True {
                  n222 = call-poly <vilib>:"Write Delimited Spreadsheet.vi"("file path (dialog if empty)"=w577, "1D data"=w575, "append to file? (new file:F)"="append csv", "delimiter (\\t)"="," ("delimiter (\\t)")) -> ()  [unwired: 10 in, 2 out]
                }
              }
              n223 = Replace Array Subset(array=w540, new element=0.0 ("new element/subarray"), index=w539) -> (w541:dbl[])
              "fine" <- w507
            }
          }
        }
      }
    }
    n224 = case shown="True" "RST" {
      tunnel: w209 -> [w311 _]
      tunnel: [w311 0] -> w237
      tunnel: [w310 w312] -> w235
      tunnel: w210 -> [w310 _]
      frame False {
      }
      frame True {
        n225 = Get Date/Time In Seconds() -> (seconds since 1Jan1904=w312:timestamp)
      }
    }
  }
  "error out 2" <- w48
  n226 = Close File(refnum=w27, error in=w88) -> (error out=→"error out":errorcluster)  [unwired: 1 out]
  n227 = call-poly <vilib>:"Write Delimited Spreadsheet.vi"("file path (dialog if empty)"=w61, "2D data"=w62, "append to file? (new file:F)"=FALSE, "transpose? (no:F)"=TRUE, "delimiter (\\t)"="," ("delimiter (\\t)")) -> ()  [unwired: 9 in, 2 out]
